vi "Image Processing-forUDP.vi"() -> ()   [LabVIEW 2016]
uses:
  <vilib>/rvi/Emulation/niFpgaGetClockAttributes.vi
  <vilib>/rvi/Emulation/niFpgaSctlEmulationGetInTimedLoop.vi
  <vilib>/rvi/Emulation/niFpgaEmulationReportErrorSimple.vi
  <vilib>/rvi/Emulation/niFpgaProcessEmulError.vi
  <vilib>/rvi/DataTransferAndStorage/Container/Common/niFpgaContainerGetUniqueNameForEmu.vi
  <vilib>/rvi/DataTransferAndStorage/Container/Common/niFpgaContainerSetEmuInfo.vi
  <vilib>/rvi/eio/common/nirviEmuReportErrorAndStop.vi
  <vilib>/rvi/eio/common/nirviEmuTemplateMethod_errors.vi
  <vilib>/rvi/interface/RandomDataEmulation/niFpgaRandomDataHandleErrors.vi
  <vilib>/rvi/Emulation/niFpgaCriticalErrorInLSC.vi
  <vilib>/rvi/LocalResourceManager/LocalResourceManager.xnode
  <vilib>/eio/EIONode/EIONode.xnode
  <vilib>/rvi/DataTransferAndStorage/Container/XNode/niFpgaContainer.xnode
  <vilib>/rvi/interface/RandomDataEmulation/nirviRandomDataFpgaReadWriteTemplate.vi
panel:
  in  "Mode LED Status":bool=TRUE
  in  "Radio LED Green":bool
  in  "readyForInput":bool
  in  "InCount":u32
  in  "picRemains":u8
  in  "OutCount":u32
  in  "setOutputType":u8=1
  out "getOutputType":u8=1
  out "DV":bool=TRUE
  out "dec deHeight":u16
  out "dec deWidth":u16
  out "dec Height":u16
  out "dec Width":u16
  out "Width":u16=320
  out "Height":u16=240
  out "deHeight":u16=240
  out "deWidth":u16=320
  out "outputExtreme2":bool=TRUE
  out "outputExtreme1":bool=TRUE
  out "outputDOG2":bool=TRUE
  out "outputDOG1":bool=TRUE
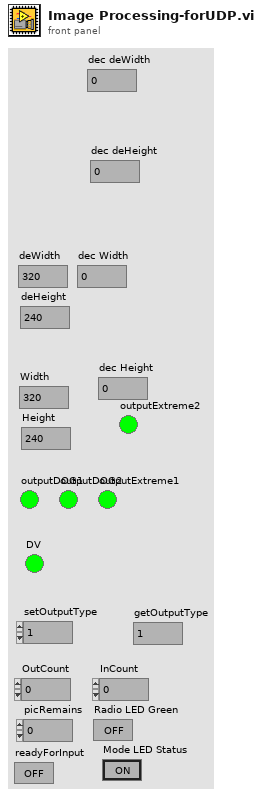
[diagram p1: front panel]
types:
  T1 = cluster{"curCol":u16, "curRow":u16, "Width":u16, "dec Height":u16, "Data Out":u8, bool}
  T2 = cluster{"curCol":u16, "curRow":u16, "Width":u16, "dec Height":u16, "GaussianFilterData out":u8, "DV out":bool}
  T3 = cluster{"t":i16, "t":i16, "deWidth":u16, "dec deHeight":u16, "GaussianFilterData out":u8, "DV out":bool}
  T4 = cluster{"t":i16, "t":i16, "deWidth":u16, "dec deHeight":u16, "Data Out":u8, "DV out":bool}
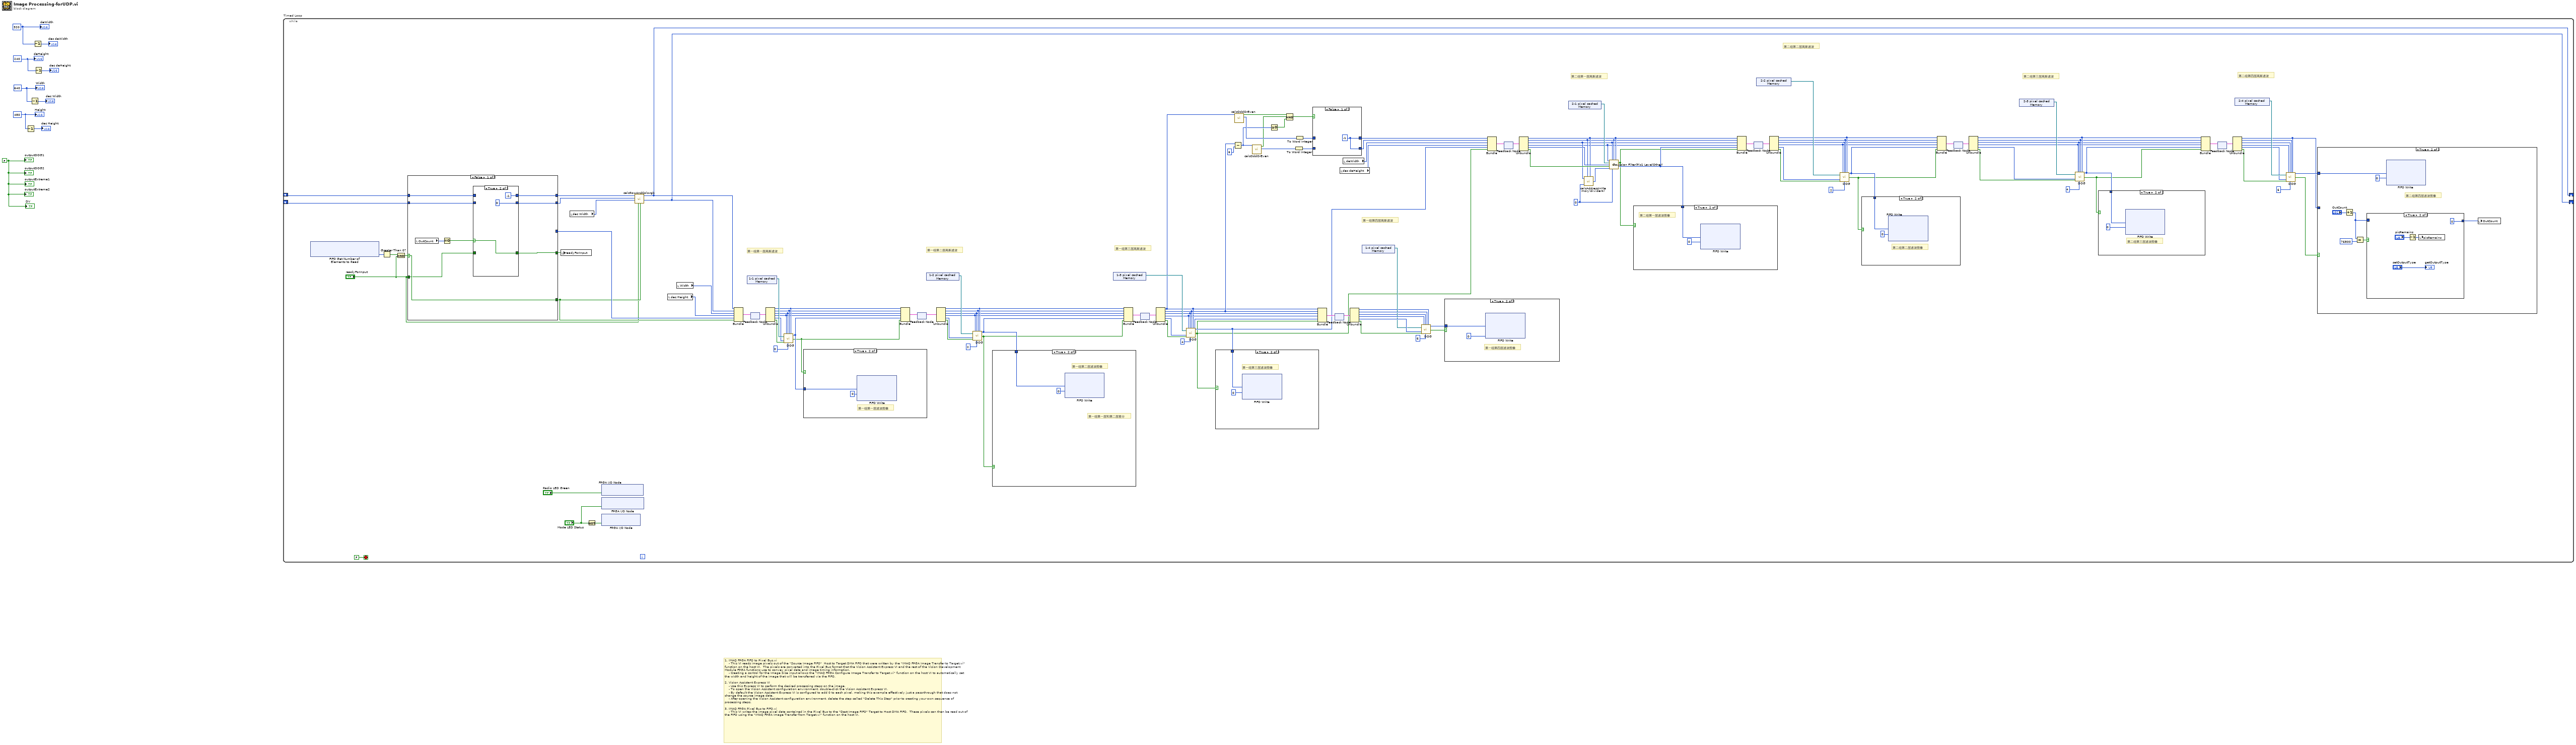
[diagram p0: block diagram]
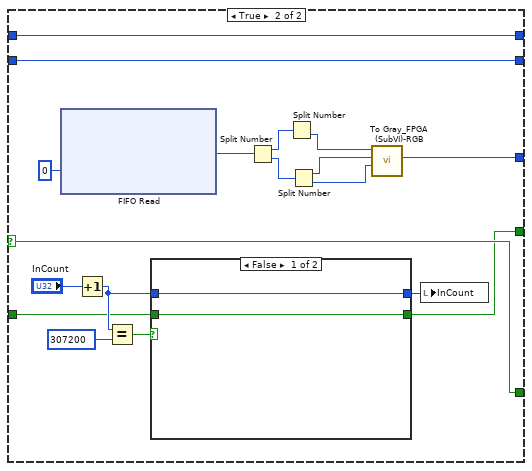
[diagram p3: hidden frame]
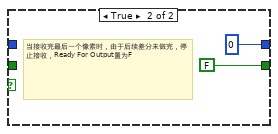
[diagram p4: hidden frame]
diagram:
  w6 = i16 480
  w9 = i16 640
  w2 = i16 240
  w4 = i16 320
  w1 = FALSE
  # "1. IMAQ FPGA FIFO to Pixel Bus.vi\n    - This VI reads image pixels out of the \"Source Image FIFO\"  Host to Target DMA FIFO that were written by the \"IMAQ FPGA Image Transfer to Target.vi\" function on the host VI.  The pixels are converted into the Pixel Bus format that the Vision Assistant Express VI and the rest of the Vision Development Module FPGA functions use to convey pixel data and image timing information.\n    - Creating a control for the Image Size input allows the \"IMAQ FPGA Configure Image Transfer to Target.vi\" function on the host VI to automatically set the width and height of the image that will be transferred via the FIFO.\n\n2. Vision Assistant Express VI\n    - Use this Express VI to perform the desired processing steps on the image.\n    - To open the Vision Assistant configuration environment, double-click the Vision Assistant Express VI.\n    - By default the Vision Assistant Express VI is configured to add 0 to each pixel, making this example effectively just a pass-through that does not change the source image data.\n    - After opening the Vision Assistant configuration environment, delete the step called \"Delete This Step\" prior to creating your own sequence of processing steps.\n\n3. IMAQ FPGA Pixel Bus to FIFO.vi\n    - This VI writes the image pixel data contained in the Pixel Bus to the \"Dest Image FIFO\" Target to Host DMA FIFO.  These pixels can then be read out of the FIFO using the \"IMAQ FPGA Image Transfer from Target.vi\" function on the host VI."
  n1 = Decrement(x=w6) -> (x-1=→"dec Height":i16)
  n2 = Decrement(x=w9) -> (x-1=→"dec Width":i16)
  n3 = Decrement(x=w4) -> (x-1=→"dec deWidth":i16)
  n4 = Decrement(x=w2) -> (x-1=→"dec deHeight":i16)
  n5 = while "Timed Loop" {
    shift-right: [w136] -> _
    shift-left: _ -> [w138]
    shift-right: [w137] -> _
    shift-left: _ -> [w139]
    stop <- FALSE stop-if-true
    w103 = u8 0 ("delayRowCount")
    # "第一组第一层高斯滤波"
    # "第一组第二层高斯滤波"
    # "第一组第三层高斯滤波"
    # "第二组第一层高斯滤波"
    # "第一组第四层高斯滤波"
    # "第二组第二层高斯滤波"
    # "第二组第三层高斯滤波"
    # "第二组第四层高斯滤波"
    n6 = xnode ("FIFO Get Number of Elements to Read")() -> ("Number of Elements to Read"=w26:u32)  [unwired: 1 in, 1 out]
    n7 = Greater Than 0?(x=w26) -> (x > 0?=w24:bool)
    n8 = And(x=w24, y="readyForInput") -> (x .and. y?=w25:bool)
    n9 = case shown="False" w25 {
      selector: w25 -> [w149 w165]
      tunnel: [_ w166] -> w85
      tunnel: [w149 w165] -> w23
      tunnel: [w147 w159] -> w21
      tunnel: "readyForInput" -> [w146 w158]
      tunnel: w139 -> [w145 w157]
      tunnel: [w143 w157] -> w19
      tunnel: [w142 w156] -> w18
      tunnel: w138 -> [w144 w156]
      frame False {
        n10 = local read "OutCount"() -> (w148:u32)
        n11 = Equal To 0?(x=w148) -> (x = 0?=w141:bool)
        n12 = case shown="True" w141 {
          selector: w141 -> [_ w155]
          tunnel: [w150 w155] -> w147
          tunnel: w146 -> [w150 _]
          tunnel: w145 -> [w152 _]
          tunnel: w144 -> [w151 _]
          tunnel: [w152 i16 -1] -> w143
          tunnel: [w151 i16 0] -> w142
          frame False {
          }
          frame True {
          }
        }
      }
      frame True {
        n13 = xnode ("FIFO Read")("Timeout"=0) -> ("Element"=w173:u32)  [unwired: 1 in, 2 out]
        n14 = Increment(x="InCount") -> (x+1=w160:u32)
        n15 = Equal?(x=w160, y=u32 307200) -> (x = y?=w164:bool)
        n16 = case shown="False" w164 {
          tunnel: [w175 i16 0] -> w161
          tunnel: w160 -> [w175 _]
          tunnel: [w174 FALSE ("Ready For Output")] -> w159
          tunnel: w158 -> [w174 _]
          frame False {
          }
          frame True {
            # "当接收完最后一个像素时，由于后续差分未做完，停止接收，Ready For Output置为F"
          }
        }
        n17 = Split Number(x=w173) -> (hi(x)=w171:u16, lo(x)=w172:u16)
        n18 = Split Number(x=w171) -> (lo(x)=w170:u8)  [unwired: 1 out]
        n19 = Split Number(x=w172) -> (hi(x)=w169:u8, lo(x)=w168:u8)
        n20 = call "To Gray_FPGA (SubVI)-RGB.vi"("B"=w168, "G"=w169, "R"=w170) -> ("Data Out"=w166:u8)  [unwired: 8 in]
        n21 = local write "InCount"(w161) -> ()
      }
    }
    n22 = local write "readyForInput"(w21) -> ()
    n23 = local read "dec Width"() -> (w22:u16)
    n24 = Not(x="Mode LED Status") -> (.not. x?=w27:bool)
    n25 = xnode "FPGA I/O Node"("Radio LED Green"="Radio LED Green") -> ()  [unwired: 1 in, 1 out]
    n26 = xnode "FPGA I/O Node"("Mode LED Green"="Mode LED Status") -> ()  [unwired: 1 in, 1 out]
    n27 = xnode "FPGA I/O Node"("Mode LED Red"=w27) -> ()  [unwired: 1 in, 1 out]
    n28 = call "calcRowAndCols-rgb.vi"("DV"=w23, "Ready For Input"="readyForInput", "decWidth"=w22, "preRow"=w18, "preCol"=w19) -> ("curRow"=w136:u16, "curCol"=w137:u16)  [unwired: 5 in]
    n29 = local read "dec Height"() -> (w28:u16)
    n30 = local read "Width"() -> (w29:u16)
    n31 = Bundle("curCol"=w137, "curRow"=w136, "Width"=w29, "dec Height"=w28, "Data Out"=w85, w23) -> (w89:T1)  [unwired: 1 in]
    n32 = xnode "1-1 pixel cached Memory"() -> ("Memory Out"=w91:refnum<k21>)
    n33 = feedback #1() -> (w88:T1)  [unwired: 1 in]
    n34 = feedback-in #1(w89) -> ()
    n35 = Unbundle(w88) -> ("curCol"=w82:u16, "curRow"=w81:u16, "Width"=w80:u16, "dec Height"=w79:u16, "Data Out"=w87:u8, w86:bool)
    n36 = call "DOG.vi"("pixel cached Memory"=w91, "Data in"=w87, "DV in"=w86, "Height"=w79, "Width"=w80, "DelayRowCount"=i16 0, "Rows"=w81, "Cols"=w82) -> ("GaussianFilterData out"=w78:u8, "DV out"=w77:bool)  [unwired: 9 in, 1 out]
    n37 = case shown="True" w77 {
      tunnel: w78 -> [_ w179]
      frame False {
      }
      frame True {
        # "第一组第一层滤波图像"
        n38 = xnode ("FIFO Write")("Element"=w179, "Timeout"=0) -> ()  [unwired: 1 in, 2 out]
      }
    }
    n39 = Bundle("curCol"=w82, "curRow"=w81, "Width"=w80, "dec Height"=w79, "GaussianFilterData out"=w78, "DV out"=w77) -> (w83:T2)  [unwired: 1 in]
    n40 = feedback #2() -> (w84:T2)  [unwired: 1 in]
    n41 = feedback-in #2(w83) -> ()
    n42 = xnode "1-2 pixel cached Memory"() -> ("Memory Out"=w94:refnum<k21>)
    n43 = Unbundle(w84) -> ("curCol"=w74:u16, "curRow"=w73:u16, "Width"=w72:u16, "dec Height"=w71:u16, "GaussianFilterData out"=w93:u8, "DV out"=w92:bool)
    n44 = call "DOG.vi"("pixel cached Memory"=w94, "Data in"=w93, "DV in"=w92, "Height"=w71, "Width"=w72, "DelayRowCount"=i16 2, "Rows"=w73, "Cols"=w74) -> ("GaussianFilterData out"=w70:u8, "DV out"=w69:bool)  [unwired: 9 in, 1 out]
    n45 = case shown="True" w69 {
      tunnel: w70 -> [_ w181]
      frame False {
      }
      frame True {
        # "第一组第二层滤波图像"
        # "第一组第一层和第二层差分"
        n46 = xnode ("FIFO Write")("Element"=w181, "Timeout"=0) -> ()  [unwired: 1 in, 2 out]
      }
    }
    n47 = xnode "1-3 pixel cached Memory"() -> ("Memory Out"=w100:refnum<k21>)
    n48 = Bundle("curCol"=w74, "curRow"=w73, "Width"=w72, "dec Height"=w71, "GaussianFilterData out"=w70, "DV out"=w69) -> (w76:T2)  [unwired: 1 in]
    n49 = feedback #3() -> (w75:T2)  [unwired: 1 in]
    n50 = feedback-in #3(w76) -> ()
    n51 = Unbundle(w75) -> ("curCol"=w15:u16, "curRow"=w66:u16, "Width"=w65:u16, "dec Height"=w64:u16, "GaussianFilterData out"=w101:u8, "DV out"=w102:bool)
    n52 = call "DOG.vi"("pixel cached Memory"=w100, "Data in"=w101, "DV in"=w102, "Height"=w64, "Width"=w65, "DelayRowCount"=i16 4, "Rows"=w66, "Cols"=w15) -> ("GaussianFilterData out"=w55:u8, "DV out"=w54:bool)  [unwired: 9 in, 1 out]
    n53 = case shown="True" w54 {
      tunnel: w55 -> [_ w186]
      frame False {
      }
      frame True {
        # "第一组第三层滤波图像"
        n54 = xnode ("FIFO Write")("Element"=w186, "Timeout"=0) -> ()  [unwired: 1 in, 2 out]
      }
    }
    n55 = Subtract(x=w66, y=i16 6) -> (x-y=w12:u16)
    n56 = call "calcOddOrEven.vi"("number"=w15) -> ("outputNum"=w14:u16, "IsEven?"=w13:bool)  [unwired: 9 in]
    n57 = call "calcOddOrEven.vi"("number"=w12) -> ("outputNum"=w10:u16, "IsEven?"=w11:bool)  [unwired: 9 in]
    n58 = Greater Or Equal To 0?(x=w12) -> (x >= 0?=w97:bool)
    n59 = Compound Arithmetic op=AND(w13, w11, w97) -> (w96:bool)
    n60 = To Word Integer(number=w10) -> (16bit integer=w60:i16)
    n61 = To Word Integer(number=w14) -> (16bit integer=w61:i16)
    n62 = case shown="False" w96 {
      tunnel: [w182 w184] -> w59
      tunnel: w61 -> [_ w184]
      tunnel: [w182 w183] -> w58
      tunnel: w60 -> [_ w183]
      frame False {
        w182 = i16 -1 ("t")
      }
      frame True {
      }
    }
    n63 = Bundle("curCol"=w15, "curRow"=w66, "Width"=w65, "dec Height"=w64, "GaussianFilterData out"=w55, "DV out"=w54) -> (w67:T2)  [unwired: 1 in]
    n64 = feedback #4() -> (w68:T2)  [unwired: 1 in]
    n65 = feedback-in #4(w67) -> ()
    n66 = local read "dec deHeight"() -> (w56:u16)
    n67 = local read "deWidth"() -> (w57:u16)
    n68 = Unbundle(w68) -> ("curCol"=w105:u16, "curRow"=w115:u16, "Width"=w106:u16, "dec Height"=w114:u16, "GaussianFilterData out"=w117:u8, "DV out"=w116:bool)
    n69 = xnode "1-4 pixel cached Memory"() -> ("Memory Out"=w113:refnum<k21>)
    n70 = call "DOG.vi"("pixel cached Memory"=w113, "Data in"=w117, "DV in"=w116, "Height"=w114, "Width"=w106, "DelayRowCount"=i16 6, "Rows"=w115, "Cols"=w105) -> ("GaussianFilterData out"=w111:u8, "DV out"=w107:bool)  [unwired: 9 in, 1 out]
    n71 = case shown="True" w107 {
      tunnel: w111 -> [_ w190]
      frame False {
      }
      frame True {
        # "第一组第四层滤波图像"
        n72 = xnode ("FIFO Write")("Element"=w190, "Timeout"=0) -> ()  [unwired: 1 in, 2 out]
      }
    }
    n73 = Bundle("t"=w59, "t"=w58, "deWidth"=w57, "dec deHeight"=w56, "GaussianFilterData out"=w55, "DV out"=w54) -> (w62:T3)  [unwired: 1 in]
    n74 = feedback #5() -> (w63:T3)  [unwired: 1 in]
    n75 = feedback-in #5(w62) -> ()
    n76 = Unbundle(w63) -> ("t"=w51:i16, "t"=w50:i16, "deWidth"=w49:u16, "dec deHeight"=w48:u16, "GaussianFilterData out"=w109:u8, "DV out"=w110:bool)
    n77 = xnode "2-1 pixel cached Memory"() -> ("Memory Out"=w108:refnum<k21>)
    n78 = call "calcAddressInMemory(divider4).vi"("Width"=w49, "Rows"=w50, "delayRowCount"=w103, "Cols"=w51) -> ("addressInMemory"=w104:u16)  [unwired: 5 in]
    n79 = call "Gaussian Filter(Pic1 LevelOther).vi"("Height"=w48, "Width"=w49, "Rows"=w50, "Cols"=w51, "Memory in"=w108, "Data in"=w109, "DV in"=w110, "Address In"=w104, "DelayRowCount"=w103) -> ("DV out"=w46:bool, "Data Out"=w47:u8)  [unwired: 4 in, 1 out]
    n80 = case shown="True" w46 {
      tunnel: w47 -> [_ w188]
      frame False {
      }
      frame True {
        # "第二组第一层滤波图像"
        n81 = xnode ("FIFO Write")("Element"=w188, "Timeout"=0) -> ()  [unwired: 1 in, 2 out]
      }
    }
    n82 = Bundle("t"=w51, "t"=w50, "deWidth"=w49, "dec deHeight"=w48, "Data Out"=w47, "DV out"=w46) -> (w53:T4)  [unwired: 1 in]
    n83 = feedback #6() -> (w52:T4)  [unwired: 1 in]
    n84 = feedback-in #6(w53) -> ()
    n85 = xnode "2-2 pixel cached Memory"() -> ("Memory Out"=w120:refnum<k21>)
    n86 = Unbundle(w52) -> ("t"=w43:i16, "t"=w42:i16, "deWidth"=w41:u16, "dec deHeight"=w40:u16, "Data Out"=w119:u8, "DV out"=w118:bool)
    n87 = call "DOG.vi"("pixel cached Memory"=w120, "Data in"=w119, "DV in"=w118, "Height"=w40, "Width"=w41, "DelayRowCount"=i16 2, "Rows"=w42, "Cols"=w43) -> ("GaussianFilterData out"=w39:u8, "DV out"=w38:bool)  [unwired: 9 in, 1 out]
    n88 = case shown="True" w38 {
      tunnel: w39 -> [_ w192]
      frame False {
      }
      frame True {
        # "第二组第二层滤波图像"
        n89 = xnode ("FIFO Write")("Element"=w192, "Timeout"=0) -> ()  [unwired: 1 in, 2 out]
      }
    }
    n90 = Bundle("t"=w43, "t"=w42, "deWidth"=w41, "dec deHeight"=w40, "GaussianFilterData out"=w39, "DV out"=w38) -> (w44:T3)  [unwired: 1 in]
    n91 = feedback #7() -> (w45:T3)  [unwired: 1 in]
    n92 = feedback-in #7(w44) -> ()
    n93 = Unbundle(w45) -> ("t"=w35:i16, "t"=w34:i16, "deWidth"=w33:u16, "dec deHeight"=w32:u16, "GaussianFilterData out"=w123:u8, "DV out"=w122:bool)
    n94 = xnode "2-3 pixel cached Memory"() -> ("Memory Out"=w124:refnum<k21>)
    n95 = call "DOG.vi"("pixel cached Memory"=w124, "Data in"=w123, "DV in"=w122, "Height"=w32, "Width"=w33, "DelayRowCount"=i16 4, "Rows"=w34, "Cols"=w35) -> ("GaussianFilterData out"=w31:u8, "DV out"=w30:bool)  [unwired: 9 in, 1 out]
    n96 = case shown="True" w30 {
      tunnel: w31 -> [_ w194]
      frame False {
      }
      frame True {
        # "第二组第三层滤波图像"
        n97 = xnode ("FIFO Write")("Element"=w194, "Timeout"=0) -> ()  [unwired: 1 in, 2 out]
      }
    }
    n98 = Bundle("t"=w35, "t"=w34, "deWidth"=w33, "dec deHeight"=w32, "GaussianFilterData out"=w31, "DV out"=w30) -> (w36:T3)  [unwired: 1 in]
    n99 = feedback #8() -> (w37:T3)  [unwired: 1 in]
    n100 = feedback-in #8(w36) -> ()
    n101 = Unbundle(w37) -> ("t"=w127:i16, "t"=w126:i16, "deWidth"=w128:u16, "dec deHeight"=w131:u16, "GaussianFilterData out"=w133:u8, "DV out"=w132:bool)
    n102 = xnode "2-4 pixel cached Memory"() -> ("Memory Out"=w134:refnum<k21>)
    n103 = call "DOG.vi"("pixel cached Memory"=w134, "Data in"=w133, "DV in"=w132, "Height"=w131, "Width"=w128, "DelayRowCount"=i16 6, "Rows"=w126, "Cols"=w127) -> ("GaussianFilterData out"=w129:u8, "DV out"=w130:bool)  [unwired: 9 in, 1 out]
    n104 = case shown="True" w130 {
      tunnel: w129 -> [_ w201]
      tunnel: w127 -> [_ _]
      frame False {
      }
      frame True {
        # "第二组第四层滤波图像"
        n105 = Increment(x="OutCount") -> (x+1=w197:u32)
        n106 = Equal?(x=w197, y=u32 76800) -> (x = y?=w200:bool)
        n107 = case shown="True" w200 {
          tunnel: [w202 i16 0] -> w196
          tunnel: w197 -> [w202 _]
          frame False {
          }
          frame True {
            n108 = Decrement(x="picRemains") -> (x-1=w206:u8)
            n109 = local write "picRemains"(w206) -> ()
            "getOutputType" <- "setOutputType"
          }
        }
        n110 = xnode ("FIFO Write")("Element"=w201, "Timeout"=0) -> ()  [unwired: 1 in, 2 out]
        n111 = local write "OutCount"(w196) -> ()
      }
    }
  }
  "outputDOG1" <- w1
  "outputDOG2" <- w1
  "outputExtreme1" <- w1
  "outputExtreme2" <- w1
  "deWidth" <- w4
  "deHeight" <- w2
  "Width" <- w9
  "Height" <- w6
  "DV" <- w1
